vi "Is Naughty Func.vi"(7 "Disallowed Functions":string[](array[string]), 10 "GObj Refnum":refnum<vi>) -> (1 "Function":string, 2 "Naughty Function":bool, 5 "Is Func":bool)   [LabVIEW 2020, in "SoL Inspector.lvlib"]
uses:
  SoL Inspector.lvlib
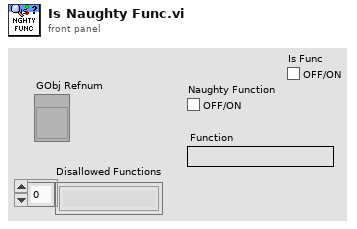
[diagram p1: front panel]
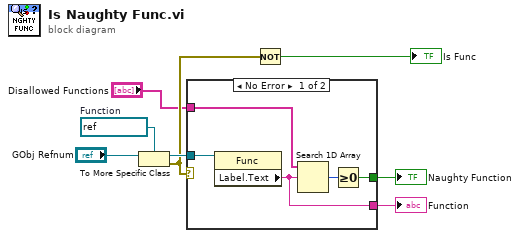
[diagram p0: block diagram]
diagram:
  w5 = refnum<vi> refnum  # Function
  n1 = To More Specific Class(target class=w5, reference="GObj Refnum") -> (specific class reference=w6:refnum<vi>, error out=w3:errorcluster)  [unwired: 1 in]
  n2 = case shown="No Error" w3 {
    tunnel: "Disallowed Functions" -> [w13 _]
    tunnel: [w11 _] -> w8
    tunnel: w6 -> [w10 _]
    tunnel: [w9 _] -> w4
    frame No Error {
      n3 = property class="Func"(reference=w10) -> ("Label.Text"=w9:string)  [unwired: 1 in, 2 out]
      n4 = Search 1D Array(1D array=w13, element=w9) -> (index of element=w12:i32)  [unwired: 1 in]
      n5 = Greater Or Equal To 0?(x=w12) -> (x >= 0?=w11:bool)
    }
    frame Error {
    }
  }
  "Naughty Function" <- w8
  "Function" <- w4
  n6 = Not(x=w3) -> (.not. x?=→"Is Func":bool)
